vi "Unflatten Path.vi"(11 "Tag value":string) -> (3 "Path":path)   [LabVIEW 2020, in "NI_VIAn_XML Parsing.lvlib"]
uses:
  <vilib>/addons/analyzer/XML Parsing/NI_VIAn_XML Parsing.lvlib
  <vilib>/addons/analyzer/VIAnCFGDataStructure/Tree Manager/API/Generate Hash.vi
  <vilib>/addons/analyzer/VIAnCFGDataStructure/Tree Manager/Tree.lvclass
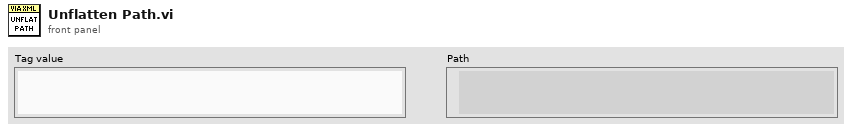
[diagram p1: front panel]
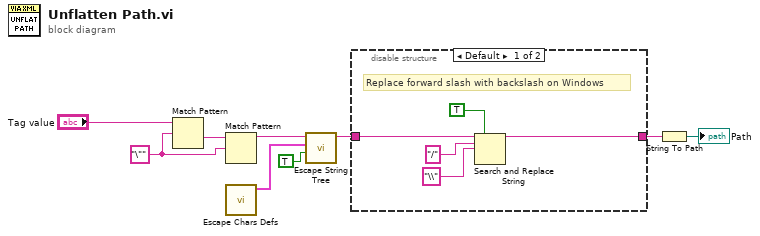
[diagram p0: block diagram]
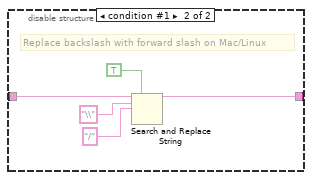
[diagram p2: hidden frame]
diagram:
  w4 = "\"" ("regular expression")
  n1 = Match Pattern(string="Tag value", regular expression=w4) -> (after substring=w3:string)  [unwired: 1 in, 3 out]
  n2 = Match Pattern(string=w3, regular expression=w4) -> (before substring=w6:string)  [unwired: 1 in, 3 out]
  n3 = call <vilib>:"Escape Chars Defs.vi"() -> ("Escapes"=w5:cluster{"String":string, "Escape":string}[])  [unwired: 11 in]
  n4 = call <vilib>:"Escape String Tree.vi"("Reverse? (False)"=TRUE, "Escapes"=w5, "String In"=w6) -> ("String Out"=w2:string)  [unwired: 8 in]
  n5 = disable-structure shown="Default" {
    disable-tunnel: w2 -> [w11 w19]
    disable-tunnel: [w10 w18] -> w1
    frame condition #0 (active) {
      # "Replace forward slash with backslash on Windows"
      n6 = Search and Replace String(replace all?=TRUE ("replace all? (F)"), input string=w11, search string="/", replace string="\\" ("search string")) -> (result string=w10:string)  [unwired: 4 in, 3 out]
    }
    frame condition #1 {
      # "Replace backslash with forward slash on Mac/Linux"
      n7 = Search and Replace String(replace all?=TRUE ("replace all? (F)"), input string=w19, search string="\\", replace string="/" ("search string")) -> (result string=w18:string)  [unwired: 4 in, 3 out]
    }
  }
  n8 = String To Path(string=w1) -> (path=→"Path":path)
